vi "AverageLiveSpectra.vi"(6 "Magnitude Averages":u8(slide) scale=1.0..10.0, 9 "old reading":waveform(dbl)[](graph), 10 "new reading":waveform(dbl)[](graph), 11 "Settings":T1 {"Ch_2" min=1 step=1; "Ch_1" min=1 max=100 step=1; "Trigger" items=["Hammer (force)", "Self-tap", "Spacebar"]; "Bandwidth" items=["1 kHz"=1, "5 kHz"=5, "10 kHz"=10, "25 kHz"=25, "50 kHz"=50, "100 kHz"=100]; "High Pass" items=["Off", "13 Hz", "104 Hz"]; "Range" items=["10 mm/s"=1, "20 mm/s"=2, "50 mm/s"=5, "100 mm/s"=10, "200 mm/s"=20, "500 mm/s"=50, "1 m/s"=100, "2 m/s"=200]; "Output" items=["Accelerometer", "Speed (from acceleration)", "Microphone", "Vibrometer", "Piezo"]; "Voltage Cal" format="%#_13g"; "Ch2 Gain" format="%#_13g"; "Ch1 Gain" format="%#_13g"; "Double bounce" min=0.0; "Mic cutoff" min=0.0 format="%#_4g"; "Hammer cutoff" min=0.0 format="%#_4g"; "Freq resolution" min=0.0; "Pre-trigger (s)" format="%#_13g"; "Date" format="%<%H:%M\n%d/%m/%y>T"; "resolution" items=["16 bit"=16, "24 bit"=24, "32 bit"=32]; "Sampling rate" items=["22050 samp/s"=22050, "44100 samp/s"=44100, "48000 samp/s"=48000]}) -> (0 "Hammer":waveform(dbl)(graph), 1 "FIFO out":waveform(dbl)[](array[waveform]), 2 "average spectrum":waveform(dbl), 3 "Power Spectrum":waveform(dbl)(graph), 4 "Microphone":waveform(dbl)(graph), 5 "Cal Hammer":waveform(dbl)[](graph), 7 "cal Mic":waveform(dbl)[](graph))   [LabVIEW 2022 SP3]
uses:
  <vilib>/Analysis/NI_AALPro.lvlib
  PreferencesControl.ctl
panel:
  out "Ch 1":waveform(dbl)(graph)
  # "Hz"
  # "dB"
  # "dB"
  # "sec"
  # "sec"
  # "mV/Pa"
  # "mV/m/s2"
  # "mV/mm/s"
  # "V/N"
  # "sec"
  # "sec"
  # "mV/N"
  # "%"
  # "%"
  # "sec"
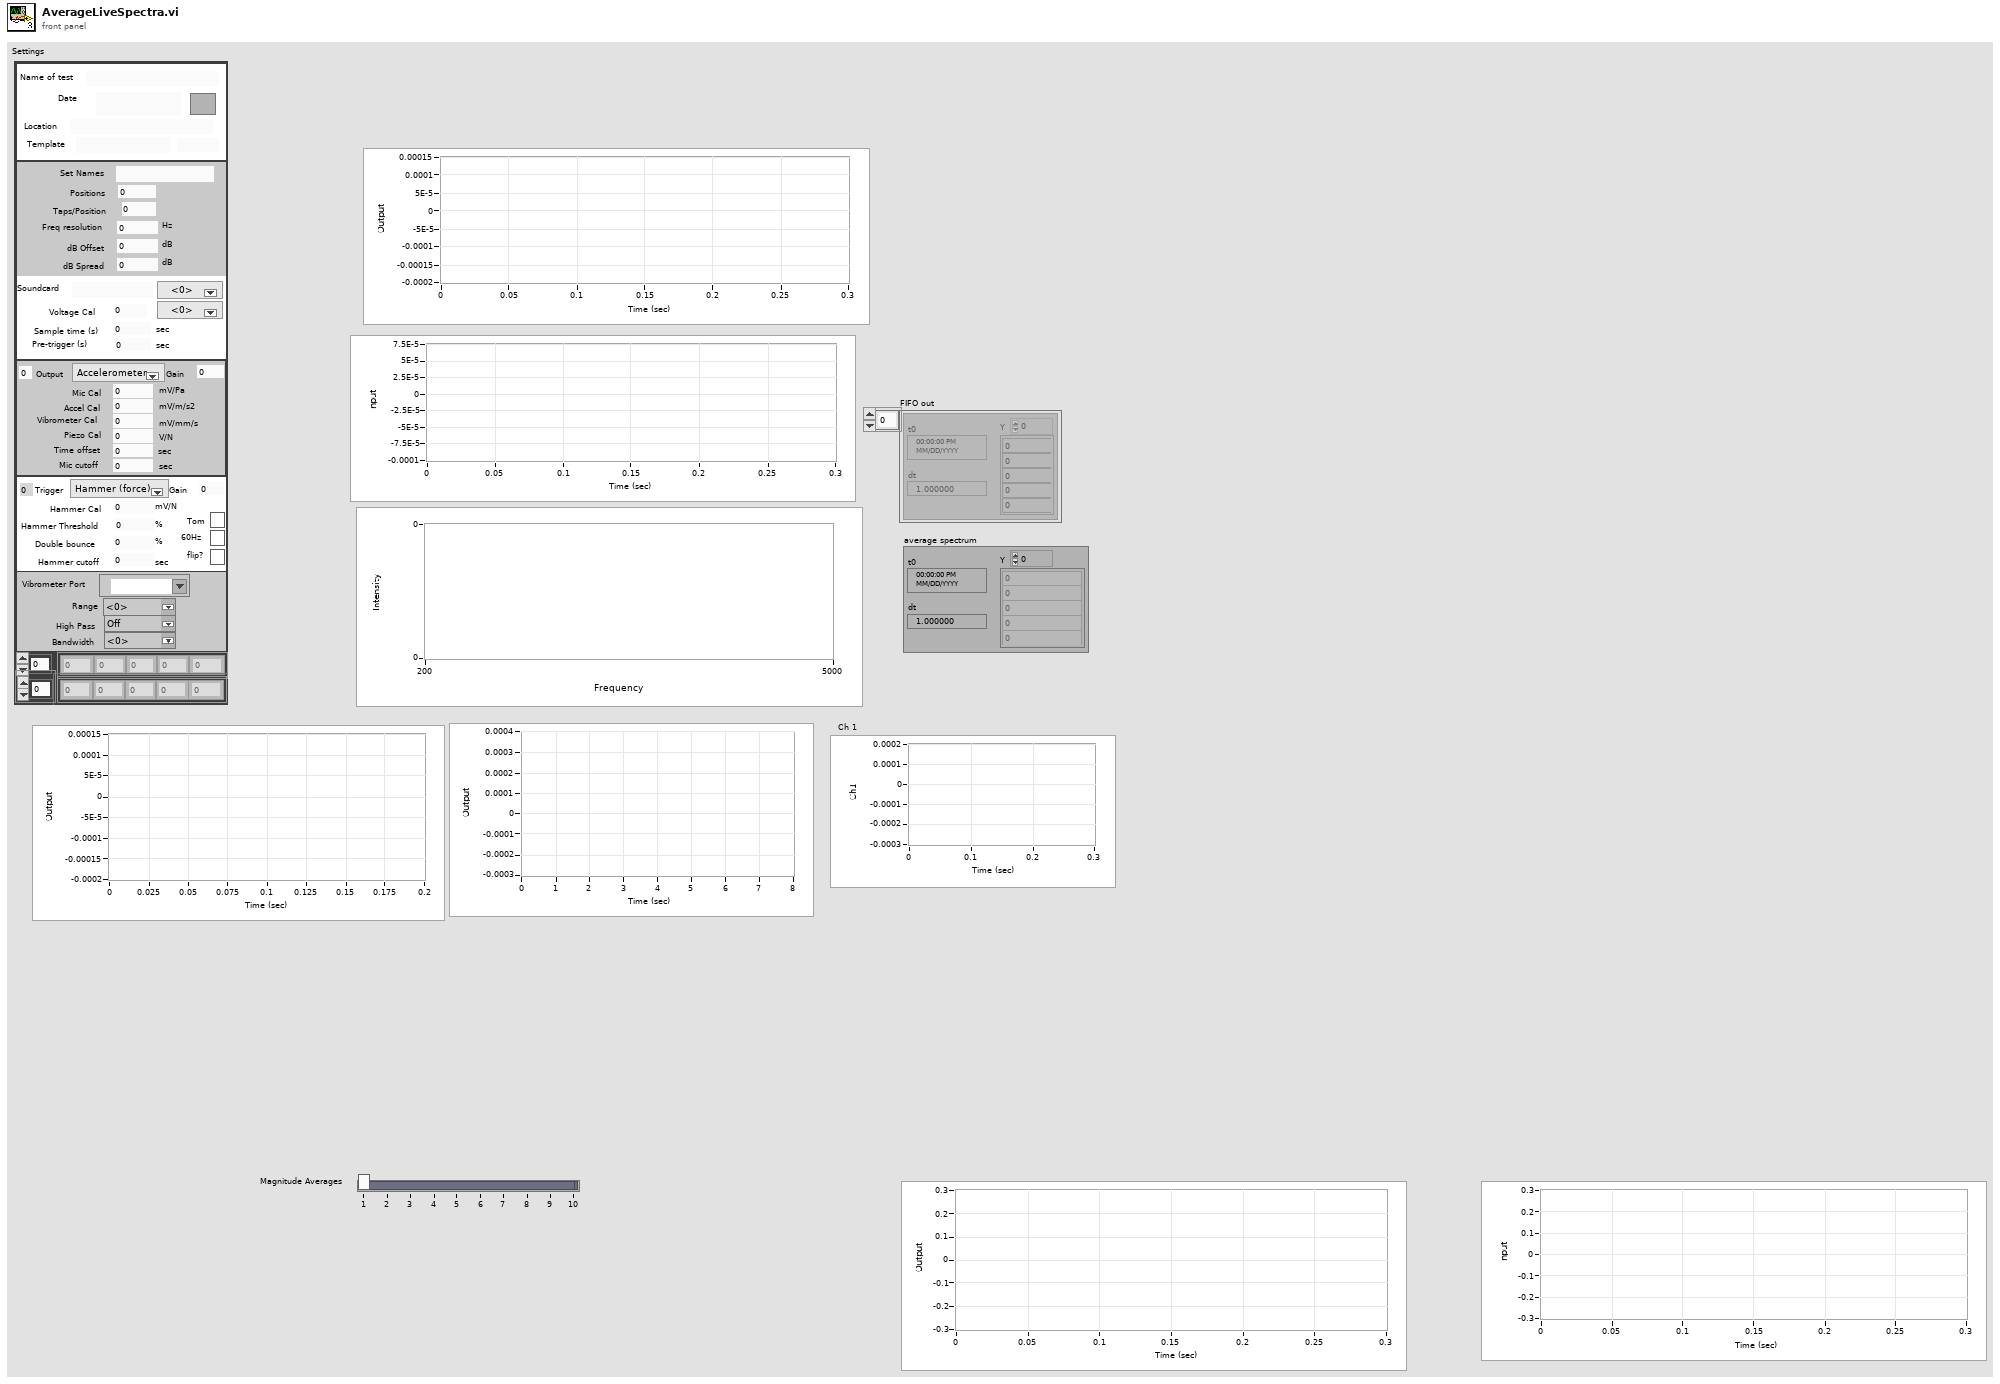
[diagram p1: front panel]
types:
  T1 = typedef "PreferencesControl.ctl" = cluster{"Name of test":string, "Date":timestamp, "Location":string, "Template":string, "Soundcard":string, "resolution":u16, "Sampling rate":u16, "Ch1 Gain ":dbl, "Ch2 Gain":dbl, "Sample time (s)":dbl, "Pre-trigger (s)":dbl, "Hammer Threshold":dbl, "Positions":i16, "Taps/Position":i16, "Set Names":string, "Freq resolution":dbl, "Hammer cutoff":dbl, "Mic cutoff":dbl, "Double bounce ":dbl, "Hammer Cal":dbl, "dB Offset":dbl, "Accel Cal":dbl, "Vibrometer Cal":dbl, "Mic Cal":dbl, "Output":u16, "Voltage Cal":dbl, "Vibrometer Port":refnum<visa-resource-name>, "Range":u16, "High Pass":u16, "Bandwidth":u16, "X Range":cluster{"Minimum":dbl, "Maximum":dbl, "Increment":dbl, "Minor Increment":dbl, "Start":dbl}[], "Y Range":cluster{"Minimum":dbl, "Maximum":dbl, "Increment":dbl, "Minor Increment":dbl, "Start":dbl}[], "dB Spread":dbl, "Trigger":u16, "Ch_1":u8, "Ch_2":u8, "flip?":bool, "60Hz":bool, "Time offset":dbl, "Piezo Cal":dbl, "Default Notes":string, "Tom":bool}
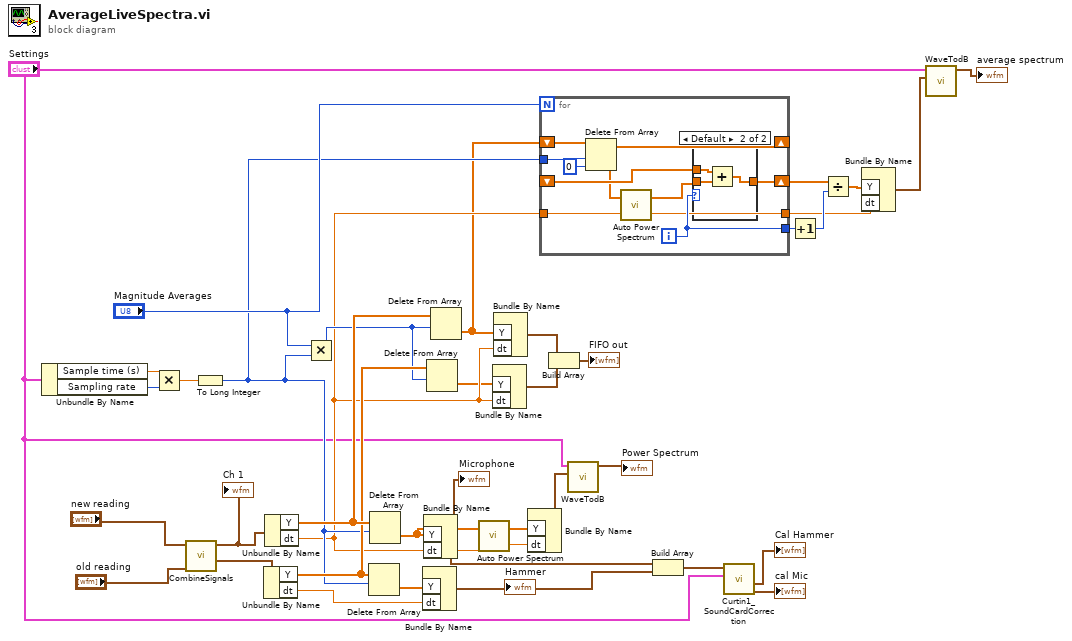
[diagram p0: block diagram]
diagram:
  n1 = Unbundle By Name("Settings") -> ("Sample time (s)"=w35:dbl, "Sampling rate"=w34:u16)
  n2 = Multiply(x=w35, y=w34) -> (x*y=w33:dbl)
  n3 = call "CombineSignals.vi"("Old signal"="old reading", "New signal"="new reading") -> ("Ch 2"=w8:waveform(dbl), "Ch 1"=w9:waveform(dbl))  [unwired: 8 in]
  "Ch 1" <- w9
  n4 = To Long Integer(number=w33) -> (32bit integer=w17:i32)
  n5 = Unbundle By Name(w8) -> ("Y"=w23:dbl[], "dt"=w29:dbl)
  n6 = Unbundle By Name(w9) -> ("Y"=w24:dbl[], "dt"=w14:dbl)
  n7 = Multiply(x="Magnitude Averages", y=w17) -> (x*y=w22:i32)
  n8 = Delete From Array(array=w23, length=w17) -> (deleted portion=w28:dbl[])  [unwired: 1 in, 1 out]
  n9 = Delete From Array(array=w24, length=w17) -> (deleted portion=w30:dbl[])  [unwired: 1 in, 1 out]
  n10 = Bundle By Name("Y"=w28, "dt"=w29) -> (w26:waveform(dbl))  [unwired: 1 in]
  "Hammer" <- w26
  n11 = Bundle By Name("Y"=w30, "dt"=w14) -> (w27:waveform(dbl))  [unwired: 1 in]
  "Microphone" <- w27
  n12 = Delete From Array(array=w23, length=w22) -> (deleted portion=w13:dbl[])  [unwired: 1 in, 1 out]
  n13 = Delete From Array(array=w24, length=w22) -> (deleted portion=w12:dbl[])  [unwired: 1 in, 1 out]
  n14 = call <vilib>:"Auto Power Spectrum.vi"("dt"=w14, "Signal (V)"=w30) -> ("df"=w31:dbl, "Power Spectrum (V^2 rms)"=w32:dbl[])
  n15 = Bundle By Name("Y"=w13, "dt"=w14) -> (w20:waveform(dbl))  [unwired: 1 in]
  n16 = Bundle By Name("Y"=w12, "dt"=w14) -> (w21:waveform(dbl))  [unwired: 1 in]
  n17 = Bundle By Name("Y"=w32, "dt"=w31) -> (w2:waveform(dbl))  [unwired: 1 in]
  n18 = for {
    N: "Magnitude Averages" -> [_]
    shift-right: [w49] -> w38
    shift-left: _ -> [w48]
    shift-right: [w44] -> _
    shift-left: w12 -> [w47]
    tunnel: w17 -> [w46]
    tunnel: [w43] -> w16
    tunnel: w14 -> [w40]
    tunnel: [w39] -> w7
    i -> [w43]
    n19 = Delete From Array(array=w47, length=w46, index=0) -> (deleted portion=w42:dbl[], array with subset deleted=w44:dbl[])
    n20 = call <vilib>:"Auto Power Spectrum.vi"("dt"=w40, "Signal (V)"=w42) -> ("df"=w39:dbl, "Power Spectrum (V^2 rms)"=w41:dbl[])
    n21 = case shown="Default" w43 {
      tunnel: [w50 w53] -> w49
      tunnel: w41 -> [w50 w51]
      tunnel: w48 -> [_ w52]
      frame 0 {
      }
      frame Default {
        n22 = Add(x=w52, y=w51) -> (x+y=w53:dbl[])
      }
    }
  }
  n23 = Build Array(w21, w20) -> (→"FIFO out":waveform(dbl)[])
  n24 = call "WaveTodB.vi"("spectrum in"=w2, "Settings"="Settings") -> ("spectrum out"=→"Power Spectrum":waveform(dbl))  [unwired: 9 in]
  n25 = Build Array(w27, w26) -> (w25:waveform(dbl)[])
  n26 = call "Curtin1_SoundCardCorrection.vi"("Settings"="Settings", "Buffer in"=w25) -> ("Microphone"=→"cal Mic":waveform(dbl)[], "Hammer"=→"Cal Hammer":waveform(dbl)[])  [unwired: 4 in, 4 out]
  n27 = Increment(x=w16) -> (x+1=w15:i32)
  n28 = Divide(x=w38, y=w15) -> (x/y=w6:dbl[])
  n29 = Bundle By Name("Y"=w6, "dt"=w7) -> (w5:waveform(dbl))  [unwired: 1 in]
  n30 = call "WaveTodB.vi"("spectrum in"=w5, "Settings"="Settings") -> ("spectrum out"=→"average spectrum":waveform(dbl))  [unwired: 9 in]
